vi "Escape_String.vi"(1 "Input String":string) -> (0 "Escaped String":string)   [LabVIEW 2011]
doc: "This VI escapes control characters in a user-generated string that would otherwise interfere with the string-parsing routines in the Growth Sequence Editor. The escape character is a backslash. For example, an input of \"Test(\"test2\"),Test3\" (without quotes) would result in the following escaped string: \"Test\\(\\\"test2\\\"\\)\\,Test3\"."
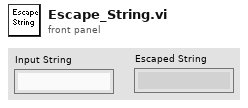
[diagram p1: front panel]
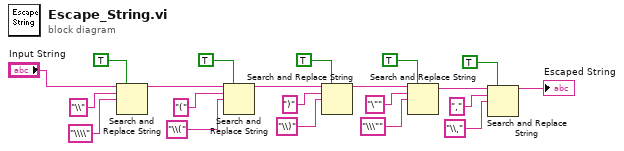
[diagram p0: block diagram]
diagram:
  n1 = Search and Replace String(replace all?=TRUE ("replace all? (F)"), input string="Input String", search string="\\", replace string="\\\\" ("replace string (\"\")")) -> (result string=w11:string)  [unwired: 4 in, 3 out]
  n2 = Search and Replace String(replace all?=TRUE ("replace all? (F)"), input string=w11, search string="(", replace string="\\(" ("replace string (\"\")")) -> (result string=w18:string)  [unwired: 4 in, 3 out]
  n3 = Search and Replace String(replace all?=TRUE ("replace all? (F)"), input string=w18, search string=")", replace string="\\)" ("replace string (\"\")")) -> (result string=w9:string)  [unwired: 4 in, 3 out]
  n4 = Search and Replace String(replace all?=TRUE ("replace all? (F)"), input string=w9, search string="\"", replace string="\\\"" ("replace string (\"\")")) -> (result string=w3:string)  [unwired: 4 in, 3 out]
  n5 = Search and Replace String(replace all?=TRUE ("replace all? (F)"), input string=w3, search string=",", replace string="\\," ("replace string (\"\")")) -> (result string=→"Escaped String":string)  [unwired: 4 in, 3 out]
